vi "Create.vi"(8 "error in (no error)":errorcluster, 11 "Database Manager":refnum<class "Database Manager.lvclass">) -> (0 "error out":errorcluster, 3 "Parent Child out":refnum<class "Parent Child.lvclass">)   [LabVIEW 2019, in "HierDAL Library.lvlib" / "Database.lvlib" / "Repositories.lvlib" / "Parent Child.lvclass"]
uses:
  Parent Child.lvclass
  Database Manager Class/Database Manager.lvclass
  Parent Child.lvclass/Parent Child.ctl
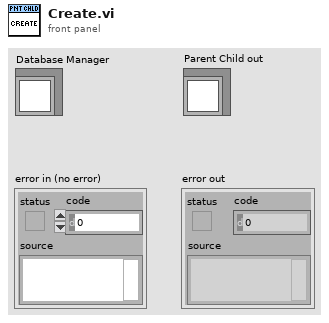
[diagram p1: front panel]
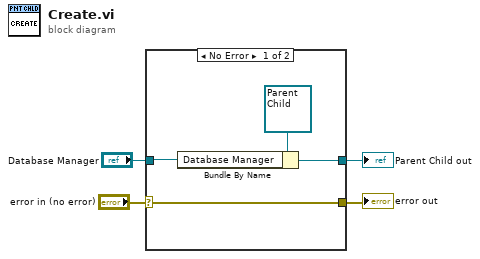
[diagram p0: block diagram]
diagram:
  n1 = case shown="No Error" "error in (no error)" {
    selector: "error in (no error)" -> [w8 w9]
    tunnel: [w8 w9] -> w1
    tunnel: [w6 _] -> w2
    tunnel: "Database Manager" -> [w7 _]
    frame No Error {
      n2 = Bundle By Name(cluster=refnum<class "Parent Child.lvclass"> refnum ("Parent Child out"), "Database Manager"=w7) -> (w6:refnum<class "Parent Child.lvclass">)
    }
    frame Error {
    }
  }
  "error out" <- w1
  "Parent Child out" <- w2
